vi "MTM2_putSample_positionIMS.vi"(8 "error in (no error)":errorcluster, 11 "positionIMS_Ctl":T1) -> (0 "error out":errorcluster, 2 "function return":i32, 3 "positionIMS_Ctl out":T1)   [LabVIEW 2018, in "SALLV_MTM2.lvlib"]
doc: "int MTM2_shm_putSample_positionIMSLV(MTM2_positionIMSLV *positionIMS_Ctl );"
uses:
  DataTypes/positionIMS.ctl
  SALLV_MTM2.lvlib
  SALLV_MTM2.so
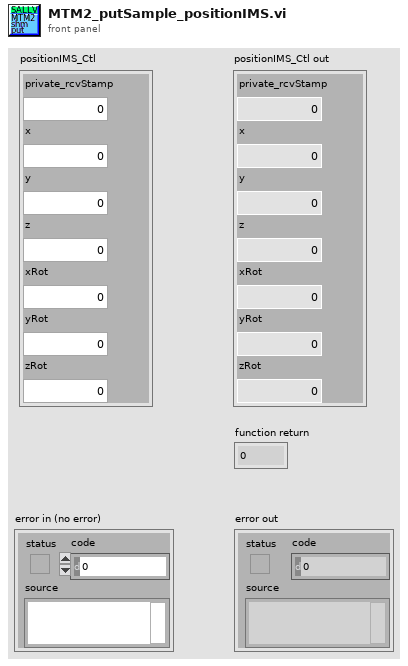
[diagram p1: front panel]
types:
  T1 = typedef "SALLV_MTM2.lvlib/positionIMS.ctl" = cluster{"private_rcvStamp":dbl, "x":dbl, "y":dbl, "z":dbl, "xRot":dbl, "yRot":dbl, "zRot":dbl}
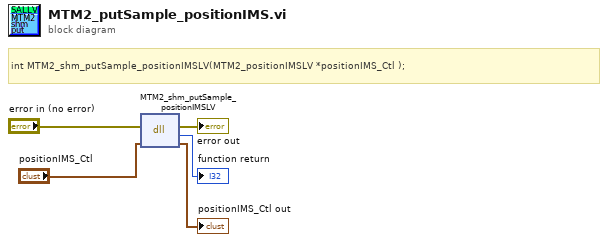
[diagram p0: block diagram]
diagram:
  # "int MTM2_shm_putSample_positionIMSLV(MTM2_positionIMSLV *positionIMS_Ctl );"
  n1 = dll-call lib="home/ttsai/Documents/salTestLabViewApi/SALLV_MTM2/SALLV_MTM2.*" fn="MTM2_shm_putSample_positionIMSLV"(error in="error in (no error)", "positionIMS_Ctl"="positionIMS_Ctl") -> (error out=→"error out":errorcluster, →"function return":i32, "positionIMS_Ctl"=→"positionIMS_Ctl out":T1)  [unwired: 2 in, 1 out]
